vi "_Write Spreadsheet.vi"(1 "Table":string[][](array[string]), 2 "Titles":string[](array[string]), 3 "Start Path":path) -> (0 "error out":errorcluster)   [LabVIEW 2012]
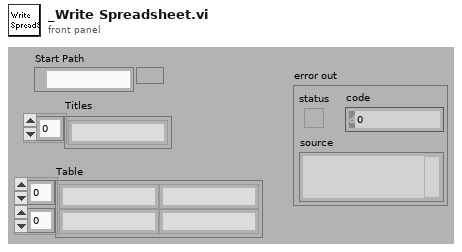
[diagram p1: front panel]
types:
  T1 = enum16{"open", "replace", "create", "open or create", "replace or create", "replace or create with confirmation"}
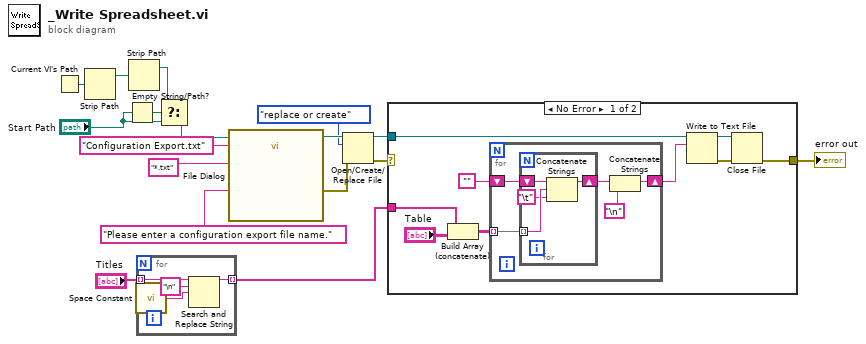
[diagram p0: block diagram]
diagram:
  n1 = Current VI's Path() -> (path=w15:path)
  n2 = Strip Path(path=w15) -> (stripped path=w16:path)  [unwired: 1 out]
  n3 = Empty String/Path?(string/path="Start Path") -> (empty?=w17:bool)
  n4 = Strip Path(path=w16) -> (stripped path=w14:path)  [unwired: 1 out]
  n5 = for {
    tunnel: "Titles" -> [w21] mode=indexing
    tunnel: [w18] -> w10 mode=indexing
    n6 = call <vilib>:"Space Constant.vi"() -> ("String"=w19:string)
    n7 = Search and Replace String(input string=w21, search string="\n", replace string=w19) -> (result string=w18:string)  [unwired: 1 in, 7 out]
  }
  n8 = Select(t=w14, s=w17, f="Start Path") -> (s? t:f=w6:path)
  n9 = call "File Dialog"("start path"=w6, "prompt"="Please enter a configuration export file name.", "default name"="Configuration Export.txt", "pattern (all files)"="*.txt" ("pattern")) -> ("selected path"=w3:path, "error out"=w2:errorcluster)  [unwired: 8 in, 2 out]
  n10 = Open/Create/Replace File(file path (use dialog)=w3, error in=w2, operation (0:open)=T1."replace or create") -> (refnum out=w4:refnum<file>, error out=w5:errorcluster)  [unwired: 3 in, 1 out]
  n11 = case shown="No Error" w5 {
    selector: w5 -> [_ w40]
    tunnel: w4 -> [w27 _]
    tunnel: [w23 w40] -> w12
    tunnel: w10 -> [w22 _]
    frame No Error {
      n12 = Build Array (concatenate)(w22, "Table") -> (w28:string[][])
      n13 = for {
        tunnel: w28 -> [w35] mode=indexing
        shift-right: [w33] -> w26
        shift-left: "" -> [w34]
        n14 = for {
          tunnel: w35 -> [w37] mode=indexing
          shift-right: [w38] -> w32
          shift-left: w34 -> [w39]
          n15 = Concatenate Strings(w39, w37, "\t") -> (w38:string)
        }
        n16 = Concatenate Strings(w32, "\n") -> (w33:string)
      }
      n17 = Write to Text File(file (use dialog)=w27, text=w26) -> (refnum out=w25:refnum<file>, error out=w24:errorcluster)  [unwired: 1 in, 2 out]
      n18 = Close File(refnum=w25, error in=w24) -> (error out=w23:errorcluster)  [unwired: 1 out]
    }
    frame Error {
    }
  }
  "error out" <- w12
